vi "Do.vi"(8 "error in (no error)":errorcluster, 11 "Add Form to Database Button in":refnum<class "Add Form to Database Button.lvclass">) -> (0 "error out":errorcluster, 3 "Add Form to Database Button out":refnum<class "Add Form to Database Button.lvclass">)   [LabVIEW 2020, in "Panel Form Controller.lvlib" / "Add Form to Database Button.lvclass"]
uses:
  Add Form to Database Button.lvclass
  Add Form to Database Button.lvclass/Add Form to Database Button.ctl
  <vilib>/ActorFramework/Message Enqueuer/Message Enqueuer.lvclass/Message Enqueuer.ctl
  <vilib>/ActorFramework/Message Enqueuer/Enqueue.vi
  Panel Form Controller Messages/Add row to database Msg/Add row to database Msg.lvclass
  C:/Program Files (x86)/National Instruments/LabVIEW 2020/vi.lib/ActorFramework/Message/Message.lvclass
  <vilib>/ActorFramework/Message Priority Queue/Priority Enqueue.vi
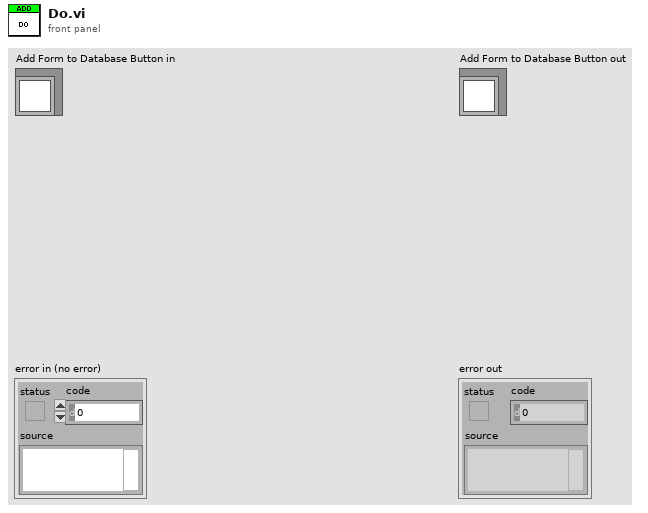
[diagram p1: front panel]
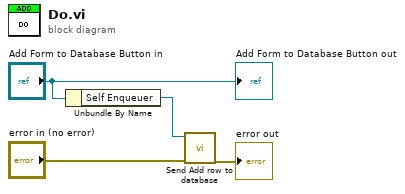
[diagram p0: block diagram]
diagram:
  n1 = Unbundle By Name("Add Form to Database Button in") -> ("Self Enqueuer"=w4:refnum<class "Message Enqueuer.lvclass">)
  n2 = call "Send Add row to database.vi"("error in (no error)"="error in (no error)", "Message Enqueuer"=w4) -> ("error out"=→"error out":errorcluster)  [unwired: 8 in, 1 out]
  "Add Form to Database Button out" <- "Add Form to Database Button in"
